vi "dialog_wait_window_multiline.vi"(8 "error in":errorcluster, 9 "parent vi reference":refnum<vi>, 10 "title":string="Please wait ...", 11 "msg":string="Please wait, generating report ...") -> (0 "error out":errorcluster)   [LabVIEW 2020, in "varilib.lvlib"]
doc: "Wait dialog window. Called by 'dialog_wait.vi'."
uses:
  varilib.lvlib
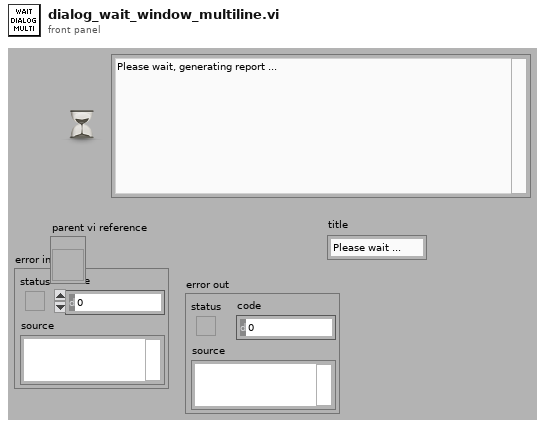
[diagram p1: front panel]
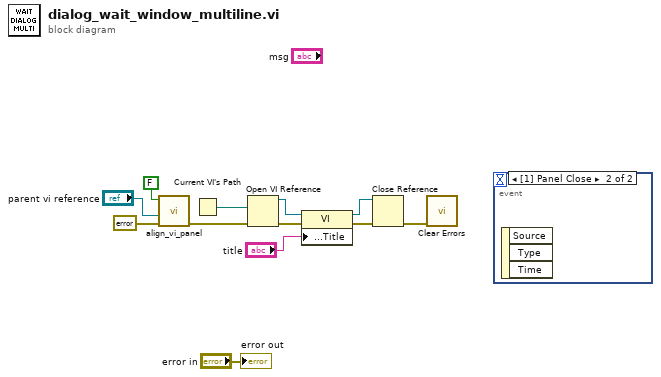
[diagram p0: block diagram]
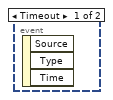
[diagram p2: hidden frame]
diagram:
  n1 = call "align_vi_panel.vi"("error in"=errorcluster {"status"=FALSE, "code"=0, "source"=""}, "ref vi reference"="parent vi reference", "use top level VI (T)"=FALSE) -> ("error out"=w4:errorcluster)  [unwired: 8 in]
  n2 = Current VI's Path() -> (path=w11:path)
  n3 = Open VI Reference(vi path=w11, error in (no error)=w4) -> (vi reference=w8:refnum<vi>, error out=w10:errorcluster)  [unwired: 4 in]
  n4 = property class="VI"(reference=w8, error in=w10, "Front Panel.Title"="title") -> (reference out=w7:refnum<vi>, error out=w9:errorcluster)
  n5 = Close Reference(reference=w7, error in (no error)=w9) -> (error out=w6:errorcluster)
  n6 = call <vilib>:"Clear Errors.vi"("error in (no error)"=w6) -> ()  [unwired: 5 in, 2 out]
  n7 = event shown="[1] Panel Close" {
    selector: _ -> [_ _]
    dyn-events: _ -> [_ _]
    timeout: _ -> [_ _]
    event Timeout {
      n8 = event-data() -> ()  [unwired: 1 in, 3 out]
    }
    event Panel Close {
      n9 = event-data() -> ()  [unwired: 1 in, 3 out]
    }
  }
  "error out" <- "error in"
